vi "5 x Lesen ErwKonfig.vi"(5 "Datenfluss (in)":bool, 8 "Fehler (Eingang, kein Fehler)":errorcluster, 9 "Factorysettings":path, 11 "appended path":path) -> (0 "Fehler (Ausgang)":errorcluster, 3 "Erw. Konfig":T8 {"Parameter Sensoren"."Druck Kalter Block" format="%#_5g"; "Parameter Sensoren"."Offset Druck FTIR IAG" format="%#_5g"; "Parameter Sensoren"."Offset Druck CG" format="%#_5g"; "Parameter Sensoren"."Offset Druck CG PMA" format="%#_5g"; "Parameter Sensoren"."Offset Durchfl.PMA" format="%#_5g"; "Parameter Sensoren"."Offset Druck Umgebung" format="%#_5g"; "Parameter Sensoren"."Offset Druck Ausgang" format="%#_5g"; "Parameter Sensoren"."Offset Durchfl.FTIR" format="%#_5g"; "Parameter Sensoren"."Kal.Durchfl.PMA" format="%.3g"; "Parameter Sensoren"."Kal.Durchfl.FTIR" format="%.3g"; "PID-Parameter Anzeige"."Heizung\nFB-Druckregler"."max. OUT" format="%#_5g"; "PID-Parameter Anzeige"."Heizung\nFB-Druckregler"."Regelzonengr." format="%#_5g"; "PID-Parameter Anzeige"."Heizung\nFB-Druckregler"."D-Anteil" format="%#_5g"; "PID-Parameter Anzeige"."Heizung\nFB-Druckregler"."I-Anteil" format="%#_5g"; "PID-Parameter Anzeige"."Heizung\nFB-Druckregler"."P-Anteil" format="%.1f"; "PID-Parameter Anzeige"."Heizleitung\nExtern"."max. OUT" format="%#_5g"; "PID-Parameter Anzeige"."Heizleitung\nExtern"."Regelzonengr." format="%#_5g"; "PID-Parameter Anzeige"."Heizleitung\nExtern"."D-Anteil" format="%#_5g"; "PID-Parameter Anzeige"."Heizleitung\nExtern"."I-Anteil" format="%#_5g"; "PID-Parameter Anzeige"."Heizleitung\nExtern"."P-Anteil" format="%.1f"; "PID-Parameter Anzeige"."Heizung\nHeizleitungen"."max. OUT" format="%#_5g"; "PID-Parameter Anzeige"."Heizung\nHeizleitungen"."Regelzonengr." format="%#_5g"; "PID-Parameter Anzeige"."Heizung\nHeizleitungen"."D-Anteil" format="%#_5g"; "PID-Parameter Anzeige"."Heizung\nHeizleitungen"."I-Anteil" format="%#_5g"; "PID-Parameter Anzeige"."Heizung\nHeizleitungen"."P-Anteil" format="%.1f"; "PID-Parameter Anzeige"."Heizung\nPumpe"."max. OUT" format="%#_5g"; "PID-Parameter Anzeige"."Heizung\nPumpe"."Regelzonengr." format="%#_5g"; "PID-Parameter Anzeige"."Heizung\nPumpe"."D-Anteil" format="%#_5g"; "PID-Parameter Anzeige"."Heizung\nPumpe"."I-Anteil" format="%#_5g"; "PID-Parameter Anzeige"."Heizung\nPumpe"."P-Anteil" format="%.1f"; "PID-Parameter Anzeige"."Heizung\nFilterblock"."max. OUT" format="%#_5g"; "PID-Parameter Anzeige"."Heizung\nFilterblock"."Regelzonengr." format="%#_5g"; "PID-Parameter Anzeige"."Heizung\nFilterblock"."D-Anteil" format="%#_5g"; "PID-Parameter Anzeige"."Heizung\nFilterblock"."I-Anteil" format="%#_5g"; "PID-Parameter Anzeige"."Heizung\nFilterblock"."P-Anteil" format="%.1f"; "Sonstige"."ext. Befüllung" items=["Deaktiviert", "Aktiviert"]; "Sonstige"."Dichtheitstest Umfang" items=["Pumpe / Filter / FT-IR / PNS", "Pumpe / Filter / FT-IR", "Filter / FT-IR", "FT-IR"]; "Sonstige"."Befüllung aktiv" items=["Deaktiviert", "Aktiviert"]}, 4 "Datenfluss (out)":bool)   [LabVIEW 2020, in "Konfig-Dateien.lvlib"]
uses:
  Konfig-Dateien.lvlib
  Seiten/Erweiterte Konfig/PID-Parameter Anzeige.ctl
  Seiten/Erweiterte Konfig/PID-Parameter.ctl
  Visualisierungs Elemente/Zahlen-Eingabefeld.ctl
  Seiten/Erweiterte Konfig/Sonstige Parameter.ctl
  Visualisierungs Elemente/Auswahlfeld.ctl
  Seiten/Log Konfig/Auswahlfeld aktiviert-deaktiviert.ctl
  Seiten/Erweiterte Konfig/Dichtheitstest Umfang.ctl
  Seiten/Erweiterte Konfig/Parameter Sensoren.ctl
  SysLog/SysLog Interface cRIO.ctl
  Seiten/Erweiterte Konfig/Erweiterte Konfig.lvlib
  Seiten/Log Konfig/LogKonfig.lvlib
  SysLog/SysLog_cRIO.lvlib
panel:
  # "sec"
  # "sec"
  # "°C"
  # "%"
  # "sec"
  # "sec"
  # "°C"
  # "%"
  # "sec"
  # "sec"
  # "°C"
  # "%"
  # "sec"
  # "sec"
  # "°C"
  # "%"
  # "sec"
  # "sec"
  # "°C"
  # "%"
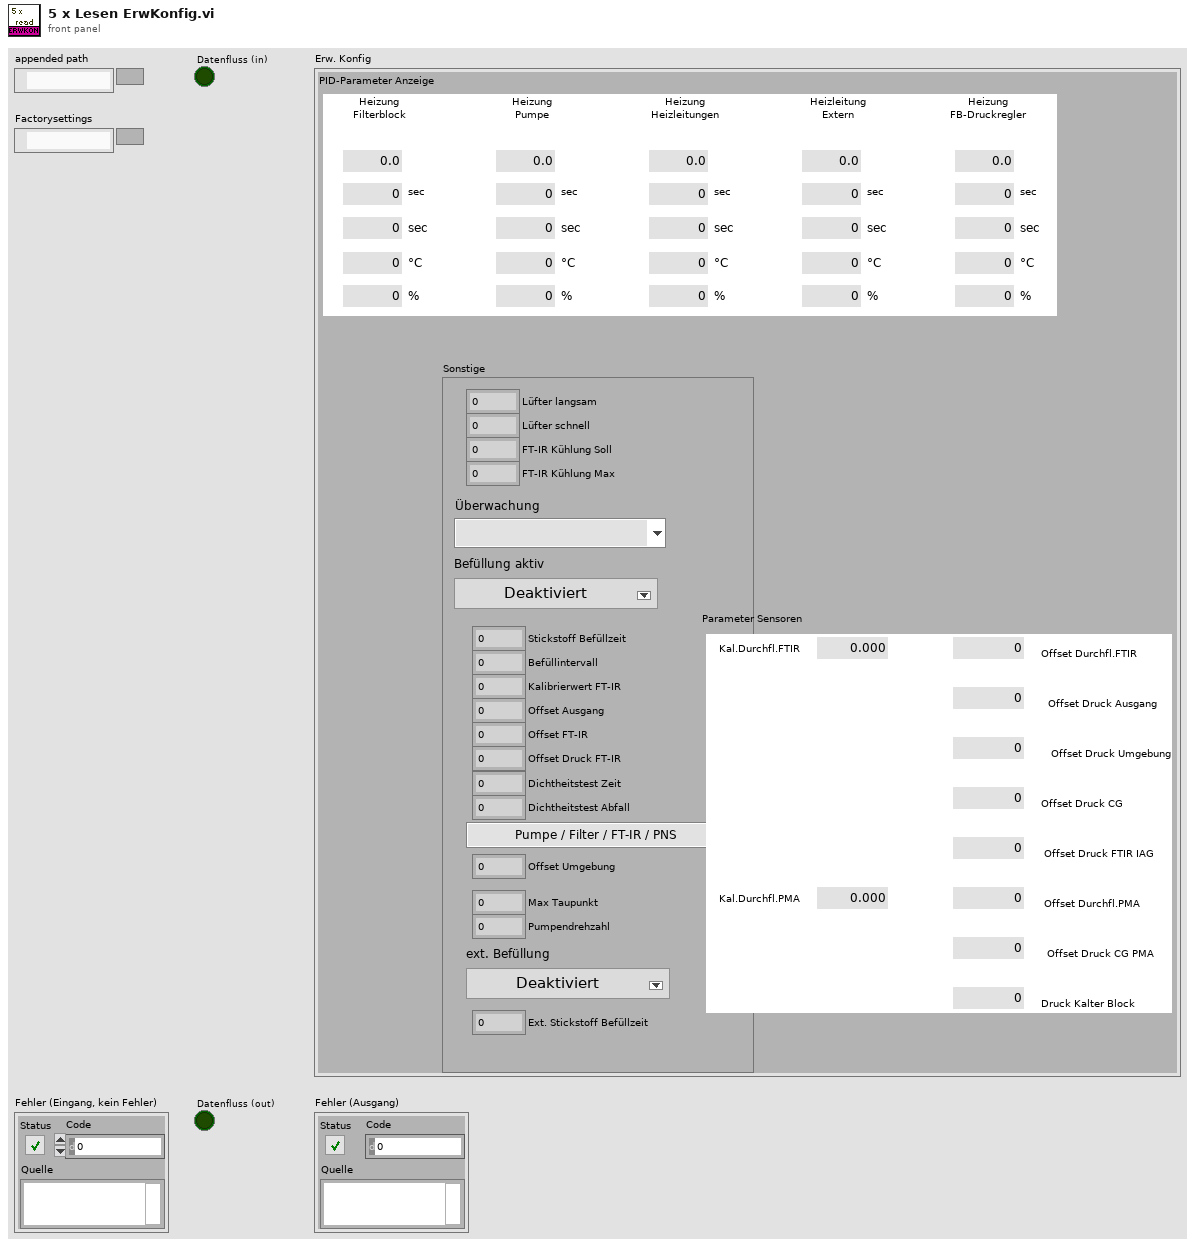
[diagram p1: front panel]
types:
  T1 = typedef "Erweiterte Konfig.lvlib/PID-Parameter Anzeige.ctl" = cluster{"Heizung\nFilterblock":T2, "Heizung\nPumpe":T2, "Heizung\nHeizleitungen":T2, "Heizleitung\nExtern":T2, "Heizung\nFB-Druckregler":T2}
  T2 = typedef "Erweiterte Konfig.lvlib/PID-Parameter.ctl" = cluster{"P-Anteil":T3, "I-Anteil":T3, "D-Anteil":T3, "Regelzonengr.":T3, "max. OUT":T3}
  T3 = typedef "Zahlen-Eingabefeld.ctl" = sgl
  T4 = typedef "Erweiterte Konfig.lvlib/Sonstige Parameter.ctl" = cluster{"Lüfter langsam":sgl, "Lüfter schnell":sgl, "FT-IR Kühlung Soll":sgl, "FT-IR Kühlung Max":sgl, "Überwachung":T5, "Befüllung aktiv":T6, "Stickstoff Befüllzeit":sgl, "Befüllintervall":sgl, "Kalibrierwert FT-IR":sgl, "Offset Ausgang":sgl, "Offset FT-IR":sgl, "Offset Druck FT-IR":sgl, "Dichtheitstest Zeit":sgl, "Dichtheitstest Abfall":sgl, "Dichtheitstest Umfang":T7, "Offset Umgebung":sgl, "Max Taupunkt":sgl, "Pumpendrehzahl":sgl, "ext. Befüllung":T6, "Ext. Stickstoff Befüllzeit":sgl}
  T5 = typedef "Auswahlfeld.ctl" = u16
  T6 = typedef "LogKonfig.lvlib/Auswahlfeld aktiviert-deaktiviert.ctl" = u16
  T7 = typedef "Erweiterte Konfig.lvlib/Dichtheitstest Umfang.ctl" = u16
  T8 = cluster{"PID-Parameter Anzeige":T1, "Sonstige":T4, "Parameter Sensoren":cluster{"Kal.Durchfl.FTIR":sgl, "Kal.Durchfl.PMA":sgl, "Offset Durchfl.FTIR":sgl, "Offset Druck Ausgang":sgl, "Offset Druck Umgebung":sgl, "Offset Durchfl.PMA":sgl, "Offset Druck CG PMA":sgl, "Offset Druck CG":sgl, "Offset Druck FTIR IAG":sgl, "Druck Kalter Block":sgl}}
  T9 = typedef "Erweiterte Konfig.lvlib/Parameter Sensoren.ctl" = cluster{"Kal.Durchfl.FTIR":sgl, "Kal.Durchfl.PMA":sgl, "Offset Durchfl.FTIR":sgl, "Offset Druck Ausgang":sgl, "Offset Druck Umgebung":sgl, "Offset Durchfl.PMA":sgl, "Offset Druck CG PMA":sgl, "Offset Druck CG":sgl, "Offset Druck FTIR IAG":sgl, "Druck Kalter Block":sgl}
  T10 = cluster{"PID-Parameter Anzeige":T1, "Sonstige":T4, "Parameter Sensoren":T9}
  T11 = typedef "SysLog_cRIO.lvlib/SysLog Interface cRIO.ctl" = cluster{"FehlermeldungsCode":i32, "ErfolgsmeldungsCode":i32, "ParameterListenString":string, "intern":bool}
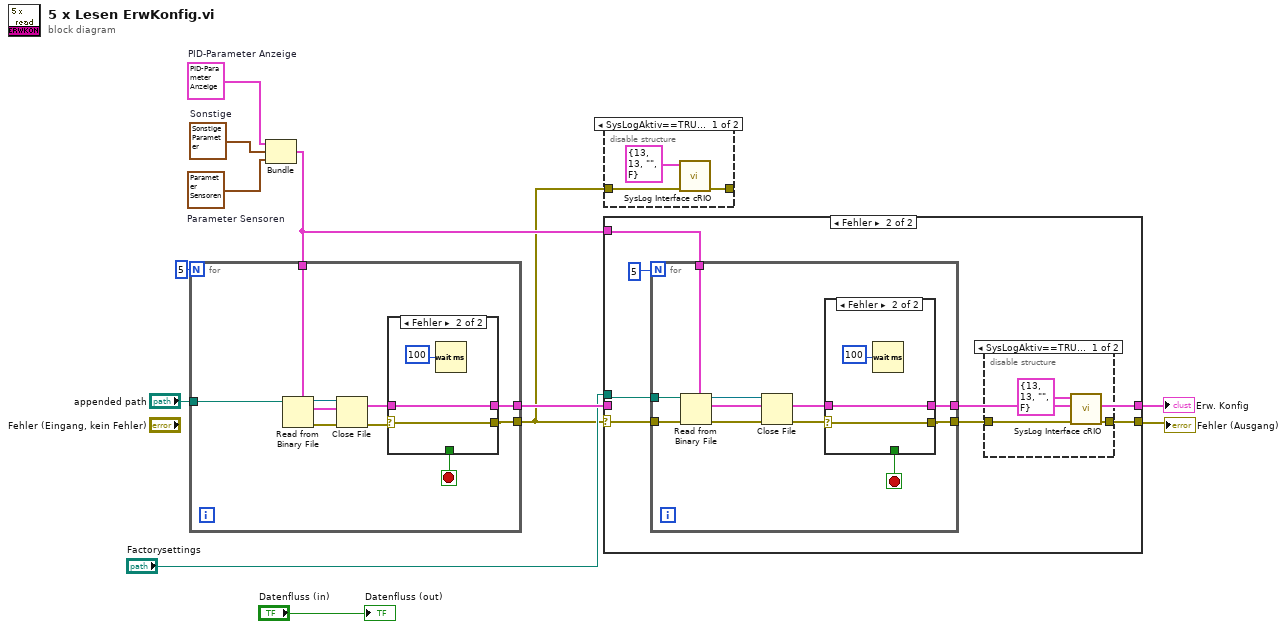
[diagram p0: block diagram]
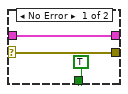
[diagram p5: hidden frame]
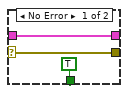
[diagram p6: hidden frame]
diagram:
  w4 = T9 {"Kal.Durchfl.FTIR"=0.0, "Kal.Durchfl.PMA"=0.0, "Offset Durchfl.FTIR"=0.0, "Offset Druck Ausgang"=0.0, "Offset Druck Umgebung"=0.0, "Offset Durchfl.PMA"=0.0, "Offset Druck CG PMA"=0.0, "Offset Druck CG"=0.0, "Offset Druck FTIR IAG"=0.0, "Druck Kalter Block"=0.0}  # Parameter Sensoren
  w5 = T4 {"Lüfter langsam"=0.0, "Lüfter schnell"=0.0, "FT-IR Kühlung Soll"=0.0, "FT-IR Kühlung Max"=0.0, "Überwachung"=0, "Befüllung aktiv"=0, "Stickstoff Befüllzeit"=0.0, "Befüllintervall"=0.0, "Kalibrierwert FT-IR"=0.0, "Offset Ausgang"=0.0, "Offset FT-IR"=0.0, "Offset Druck FT-IR"=0.0, "Dichtheitstest Zeit"=0.0, "Dichtheitstest Abfall"=0.0, "Dichtheitstest Umfang"=0, "Offset Umgebung"=0.0, "Max Taupunkt"=0.0, "Pumpendrehzahl"=0.0, "ext. Befüllung"=0, "Ext. Stickstoff Befüllzeit"=0.0}  # Sonstige
  w6 = T1 {"Heizung\nFilterblock"={"P-Anteil"=0.0, "I-Anteil"=0.0, "D-Anteil"=0.0, "Regelzonengr."=0.0, "max. OUT"=0.0}, "Heizung\nPumpe"={"P-Anteil"=0.0, "I-Anteil"=0.0, "D-Anteil"=0.0, "Regelzonengr."=0.0, "max. OUT"=0.0}, "Heizung\nHeizleitungen"={"P-Anteil"=0.0, "I-Anteil"=0.0, "D-Anteil"=0.0, "Regelzonengr."=0.0, "max. OUT"=0.0}, "Heizleitung\nExtern"={"P-Anteil"=0.0, "I-Anteil"=0.0, "D-Anteil"=0.0, "Regelzonengr."=0.0, "max. OUT"=0.0}, "Heizung\nFB-Druckregler"={"P-Anteil"=0.0, "I-Anteil"=0.0, "D-Anteil"=0.0, "Regelzonengr."=0.0, "max. OUT"=0.0}}  # PID-Parameter Anzeige
  n1 = Bundle("PID-Parameter Anzeige"=w6, "Sonstige"=w5, "Parameter Sensoren"=w4) -> (w3:T10)  [unwired: 1 in]
  n2 = for {
    N: 5 -> [_]
    tunnel: [w20] -> w9
    tunnel: "appended path" -> [w13]
    tunnel: w3 -> [w18]
    tunnel: [w14] -> w1
    stop <- w19 stop-if-true
    n3 = Read from Binary File(5:w18, 11:w13) -> (0:w16:errorcluster, 2:w21:T10, 3:w17:refnum<file>)  [unwired: 4 in, 1 out]
    n4 = Close File(refnum=w17, error in=w16) -> (error out=w15:errorcluster)  [unwired: 1 out]
    n5 = case shown="Fehler" w15 {
      selector: w15 -> [w22 w26]
      tunnel: [w22 w26] -> w14
      tunnel: w21 -> [w24 w27]
      tunnel: [w24 w27] -> w20
      tunnel: [TRUE _] -> w19
      frame No Error {
      }
      frame Error {
        n6 = Wait (ms)(milliseconds to wait=u32 100 ("Zu wartende ms")) -> ()  [unwired: 1 out]
      }
    }
  }
  n7 = case shown="Fehler" w1 {
    selector: w1 -> [w28 w31]
    tunnel: w9 -> [w29 _]
    tunnel: [w29 w36] -> w8
    tunnel: "Factorysettings" -> [_ w35]
    tunnel: w3 -> [_ w33]
    tunnel: [w28 w32] -> w2
    frame No Error {
    }
    frame Error {
      n8 = for {
        N: 5 -> [_]
        tunnel: [w48] -> w36
        tunnel: w35 -> [w50]
        tunnel: w33 -> [w46]
        tunnel: w31 -> [w42]
        tunnel: [w41] -> w30
        stop <- w47 stop-if-true
        n9 = Read from Binary File(5:w46, 8:w42, 11:w50) -> (0:w44:errorcluster, 2:w49:T10, 3:w45:refnum<file>)  [unwired: 3 in, 1 out]
        n10 = Close File(refnum=w45, error in=w44) -> (error out=w43:errorcluster)  [unwired: 1 out]
        n11 = case shown="Fehler" w43 {
          selector: w43 -> [w51 w55]
          tunnel: [w51 w55] -> w41
          tunnel: w49 -> [w53 w56]
          tunnel: [w53 w56] -> w48
          tunnel: [TRUE _] -> w47
          frame No Error {
          }
          frame Error {
            n12 = Wait (ms)(milliseconds to wait=u32 100 ("Zu wartende ms")) -> ()  [unwired: 1 out]
          }
        }
      }
      n13 = disable-structure shown="SysLogAktiv==TRUE" {
        disable-tunnel: [w38 w40] -> w32
        disable-tunnel: w30 -> [w37 w40]
        frame condition #0 (active) {
          n14 = call "SysLog Interface cRIO.vi"("Fehler (in)"=w37, "Cluster (in)"=T11 {"FehlermeldungsCode"=13, "ErfolgsmeldungsCode"=13, "ParameterListenString"="", "intern"=FALSE}) -> ("Fehler (Ausgang)"=w38:errorcluster)  [unwired: 9 in]
        }
        frame condition #1 {
        }
      }
    }
  }
  "Fehler (Ausgang)" <- w2
  "Erw. Konfig" <- w8
  n15 = disable-structure shown="SysLogAktiv==TRUE" {
    disable-tunnel: [w58 w60] -> _
    disable-tunnel: w1 -> [w57 w60]
    frame condition #0 (active) {
      n16 = call "SysLog Interface cRIO.vi"("Fehler (in)"=w57, "Cluster (in)"=T11 {"FehlermeldungsCode"=13, "ErfolgsmeldungsCode"=13, "ParameterListenString"="", "intern"=FALSE}) -> ("Fehler (Ausgang)"=w58:errorcluster)  [unwired: 9 in]
    }
    frame condition #1 {
    }
  }
  "Datenfluss (out)" <- "Datenfluss (in)"
